vi "getColor2.vi"(7 "Parâmetros Ini":T2={"Gyro Port"=0, "Sensor - Left"=3, "Sensor - Right"=2, "     Color \nSensor Port"=1, "Kp Front"=0.5, "Motor speed"=-15, "Distance to street"=0.0, "Motor speed turns"=16, "Kp Curvas"=0.0} {"Kp Front" format="%.3f"; "Color \nSensor Port" items=["Port 1", "Port 2", "Port 3", "Port 4"]; "Sensor - Right" items=["Port 1", "Port 2", "Port 3", "Port 4"]; "Sensor - Left" items=["Port 1", "Port 2", "Port 3", "Port 4"]; "Gyro Port" items=["Port 1", "Port 2", "Port 3", "Port 4"]}, 11 "NXT/EV3":T4) -> (1 "Cor":T1, 3 "NXT/EV3 2":T4)   [LabVIEW 2016]
uses:
  <vilib>/NXT/Subs/LVHSConnector.ctl
  <vilib>/NXT/LegoClasses/BrickReference/BrickReference.lvclass
  parametros.ctl
  <vilib>/NXT/Block Support/NXT_InputPort.ctl
  <vilib>/NXT/Subs/ColorSensorColors.ctl
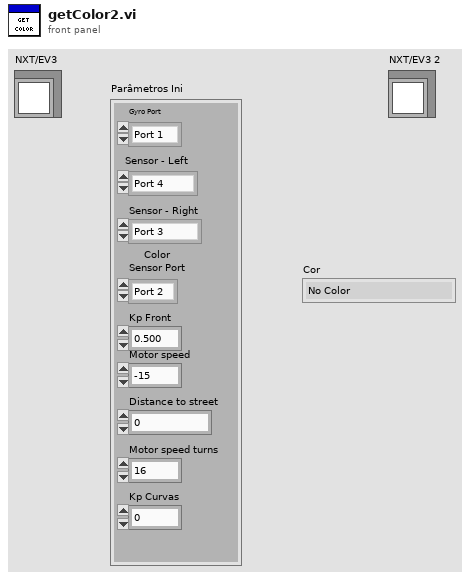
[diagram p1: front panel]
types:
  T1 = typedef "ColorSensorColors.ctl" = enum16{"No Color", "Black", "Blue", "Green", "Yellow", "Red", "White", "Brown"}
  T2 = typedef "parametros.ctl" = cluster{"Gyro Port":T3, "Sensor - Left":T3, "Sensor - Right":T3, "     Color \nSensor Port":T3, "Kp Front":dbl, "Motor speed":i32, "Distance to street":dbl, "Motor speed turns":i32, "Kp Curvas":dbl}
  T3 = typedef "NXT_InputPort.ctl" = u32
  T4 = typedef "LVHSConnector.ctl" = refnum<class "BrickReference.lvclass">
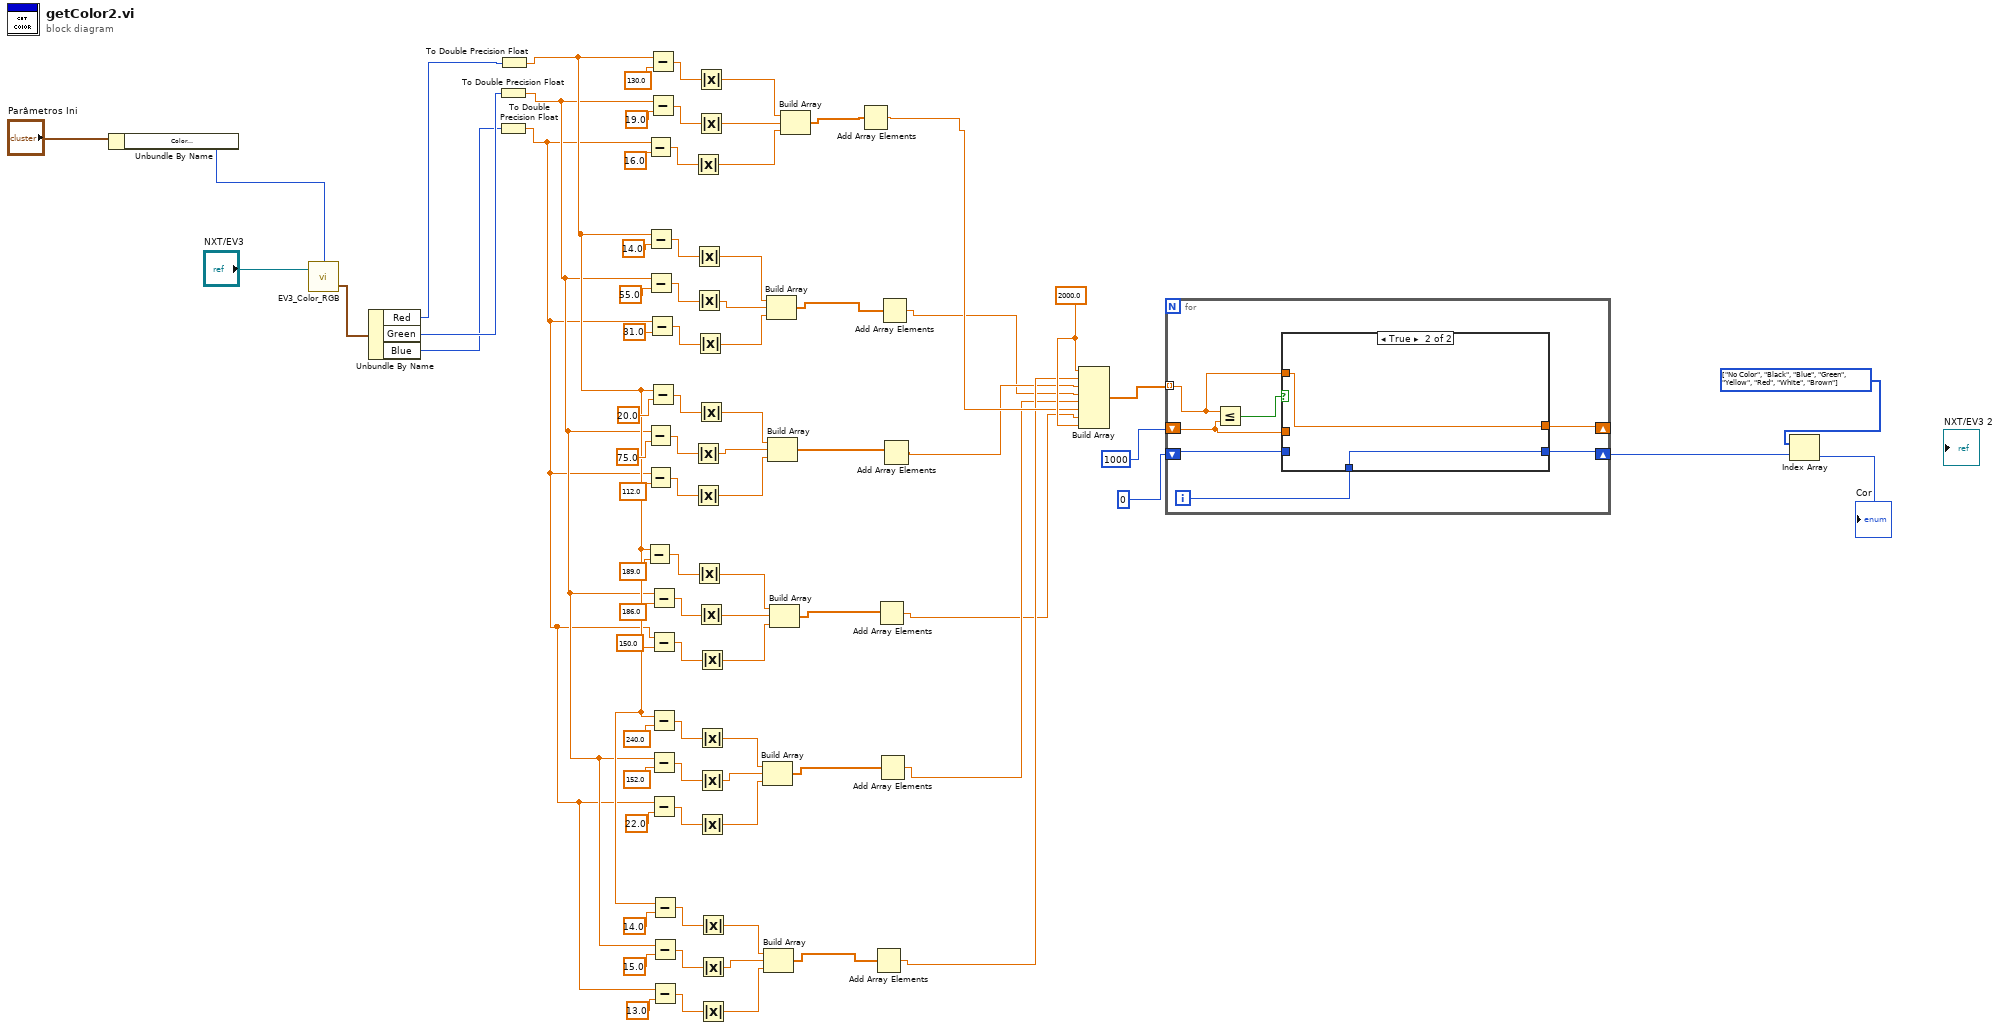
[diagram p0: block diagram]
diagram:
  w13 = 2000.0 ("element")
  w16 = T1[] [enum."No Color", enum."Black", enum."Blue", enum."Green", enum."Yellow", enum."Red", enum."White", enum."Brown"] items=["No Color", "Black", "Blue", "Green", "Yellow", "Red", "White", "Brown"]
  n1 = Unbundle By Name("Parâmetros Ini") -> ("Color \nSensor Port"=w29:T3)
  n2 = call <vilib>:"EV3_Color_RGB.vi"("NXT/EV3"="NXT/EV3", "Port (Port 1)"=w29) -> ("RGB Color"=w82:cluster{"Red":u8, "Green":u8, "Blue":u8})  [unwired: 1 in, 1 out]
  n3 = Unbundle By Name(w82) -> ("Red"=w66:u8, "Green"=w65:u8, "Blue"=w64:u8)
  n4 = To Double Precision Float(number=w65) -> (double precision float=w18:dbl)
  n5 = To Double Precision Float(number=w64) -> (double precision float=w17:dbl)
  n6 = To Double Precision Float(number=w66) -> (double precision float=w19:dbl)
  n7 = Subtract(x=w19, y=189.0) -> (x-y=w72:dbl)
  n8 = Subtract(x=w17, y=16.0) -> (x-y=w79:dbl)
  n9 = Subtract(x=w18, y=75.0) -> (x-y=w74:dbl)
  n10 = Subtract(x=w17, y=112.0) -> (x-y=w73:dbl)
  n11 = Subtract(x=w19, y=14.0) -> (x-y=w78:dbl)
  n12 = Subtract(x=w18, y=55.0) -> (x-y=w77:dbl)
  n13 = Subtract(x=w17, y=31.0) -> (x-y=w76:dbl)
  n14 = Subtract(x=w19, y=130.0) -> (x-y=w81:dbl)
  n15 = Subtract(x=w18, y=19.0) -> (x-y=w80:dbl)
  n16 = Subtract(x=w19, y=20.0) -> (x-y=w75:dbl)
  n17 = Subtract(x=w18, y=186.0) -> (x-y=w71:dbl)
  n18 = Subtract(x=w17, y=150.0) -> (x-y=w70:dbl)
  n19 = Subtract(x=w19, y=240.0) -> (x-y=w69:dbl)
  n20 = Subtract(x=w18, y=152.0) -> (x-y=w68:dbl)
  n21 = Subtract(x=w17, y=22.0) -> (x-y=w67:dbl)
  n22 = Subtract(x=w19, y=14.0) -> (x-y=w28:dbl)
  n23 = Subtract(x=w18, y=15.0) -> (x-y=w27:dbl)
  n24 = Subtract(x=w17, y=13.0) -> (x-y=w26:dbl)
  n25 = Absolute Value(x=w79) -> (abs(x)=w46:dbl)
  n26 = Absolute Value(x=w74) -> (abs(x)=w41:dbl)
  n27 = Absolute Value(x=w73) -> (abs(x)=w40:dbl)
  n28 = Absolute Value(x=w78) -> (abs(x)=w45:dbl)
  n29 = Absolute Value(x=w77) -> (abs(x)=w44:dbl)
  n30 = Absolute Value(x=w72) -> (abs(x)=w39:dbl)
  n31 = Absolute Value(x=w76) -> (abs(x)=w43:dbl)
  n32 = Absolute Value(x=w81) -> (abs(x)=w48:dbl)
  n33 = Absolute Value(x=w80) -> (abs(x)=w47:dbl)
  n34 = Absolute Value(x=w75) -> (abs(x)=w42:dbl)
  n35 = Absolute Value(x=w71) -> (abs(x)=w38:dbl)
  n36 = Absolute Value(x=w70) -> (abs(x)=w37:dbl)
  n37 = Absolute Value(x=w69) -> (abs(x)=w36:dbl)
  n38 = Absolute Value(x=w68) -> (abs(x)=w35:dbl)
  n39 = Absolute Value(x=w67) -> (abs(x)=w34:dbl)
  n40 = Absolute Value(x=w28) -> (abs(x)=w22:dbl)
  n41 = Absolute Value(x=w27) -> (abs(x)=w21:dbl)
  n42 = Absolute Value(x=w26) -> (abs(x)=w20:dbl)
  n43 = Build Array(w36, w35, w34) -> (w8:dbl[])
  n44 = Build Array(w22, w21, w20) -> (w10:dbl[])
  n45 = Build Array(w45, w44, w43) -> (w2:dbl[])
  n46 = Build Array(w42, w41, w40) -> (w4:dbl[])
  n47 = Build Array(w39, w38, w37) -> (w6:dbl[])
  n48 = Build Array(w48, w47, w46) -> (w12:dbl[])
  n49 = Add Array Elements(numeric array=w12) -> (sum=w11:dbl)
  n50 = Add Array Elements(numeric array=w10) -> (sum=w9:dbl)
  n51 = Add Array Elements(numeric array=w6) -> (sum=w5:dbl)
  n52 = Add Array Elements(numeric array=w8) -> (sum=w7:dbl)
  n53 = Add Array Elements(numeric array=w2) -> (sum=w1:dbl)
  n54 = Add Array Elements(numeric array=w4) -> (sum=w3:dbl)
  n55 = Build Array(w13, w9, w3, w1, w7, w11, w5, w13) -> (w32:dbl[])
  n56 = for {
    tunnel: w32 -> [w84] mode=indexing
    shift-right: [w89] -> _
    shift-left: 1000 -> [w88]
    shift-right: [w86] -> w15
    shift-left: 0 -> [w85]
    i -> [w87]
    n57 = Less Or Equal?(x=w84, y=w88) -> (x <= y?=w90:bool)
    n58 = case shown="True" w90 {
      tunnel: [w92 w93] -> w89
      tunnel: w88 -> [w92 _]
      tunnel: w87 -> [_ w94]
      tunnel: [w91 w94] -> w86
      tunnel: w85 -> [w91 _]
      tunnel: w84 -> [_ w93]
      frame False {
      }
      frame True {
      }
    }
  }
  n59 = Index Array(array=w16, index=w15) -> (element=→"Cor":T1)
